vi "WaitForPolytecTrigger.vi"() -> (1 "Result":string)   [LabVIEW 2020]
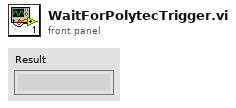
[diagram p1: front panel]
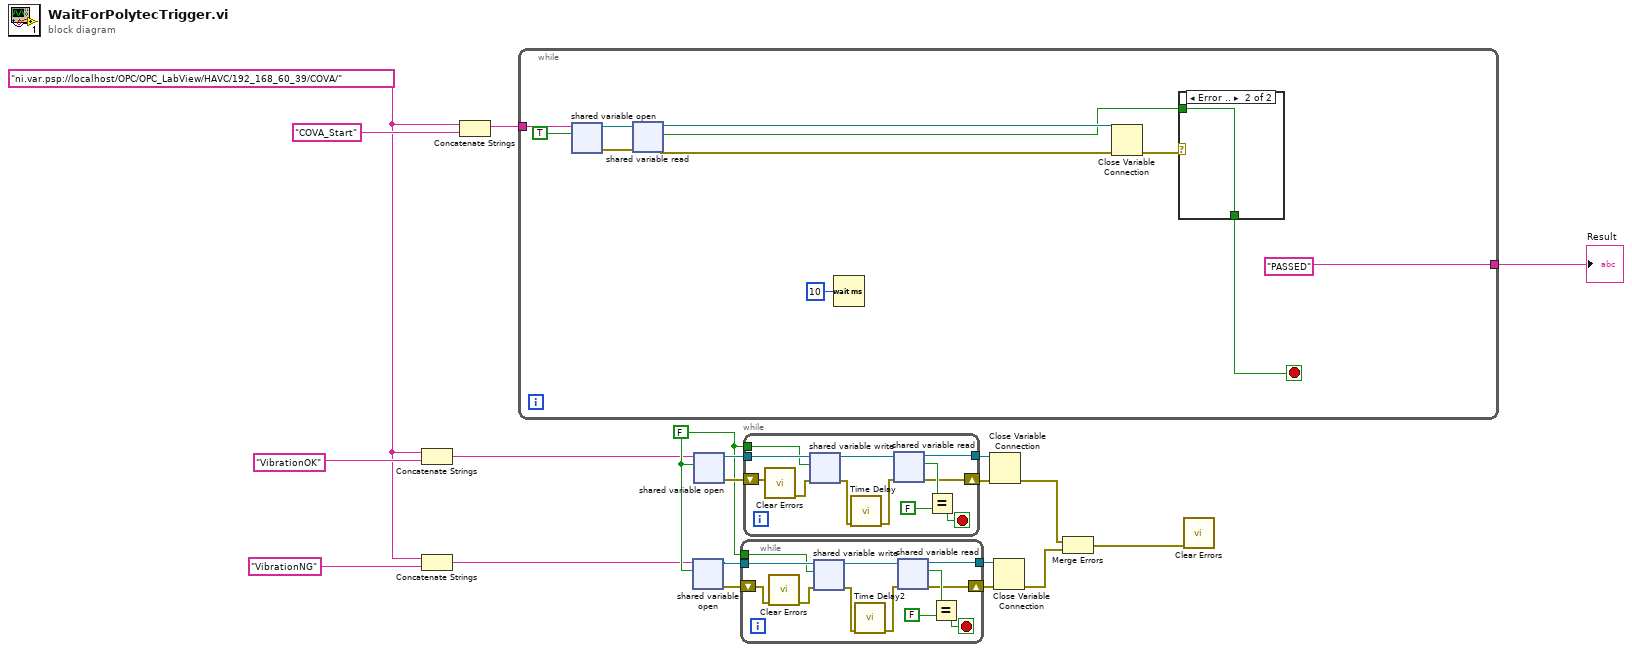
[diagram p0: block diagram]
diagram:
  w4 = FALSE
  w18 = "ni.var.psp://localhost/OPC/OPC_LabView/HAVC/192_168_60_39/COVA/" ("string")
  n1 = Concatenate Strings(w18, "VibrationOK") -> (w2:string)
  n2 = Concatenate Strings(w18, "VibrationNG" ("string")) -> (w3:string)
  n3 = Concatenate Strings(w18, "COVA_Start") -> (w16:string)
  n4 = while {
    tunnel: w16 -> [w31]
    tunnel: ["PASSED"] -> w15
    stop <- w24 stop-if-true
    n5 = shared-variable-open(w31, TRUE) -> (w28:refnum<k21>, w29:errorcluster)  [unwired: 2 in]
    n6 = shared-variable-read(w28, w29) -> (w26:refnum<k21>, w27:errorcluster, w23:bool)  [unwired: 1 out]
    n7 = Wait (ms)(milliseconds to wait=u32 10) -> ()  [unwired: 1 out]
    n8 = Close Variable Connection(8:w27, 11:w26) -> (0:w25:errorcluster)
    n9 = case shown="Error .." w25 {
      tunnel: [w32 w33] -> w24
      tunnel: w23 -> [w32 w33]
      frame No Error {
      }
      frame Error {
      }
    }
  }
  "Result" <- w15
  n10 = shared-variable-open(w3, w4) -> (w11:refnum<k21>, w12:errorcluster)  [unwired: 2 in]
  n11 = shared-variable-open(w2, w4) -> (w7:refnum<k21>, w14:errorcluster)  [unwired: 2 in]
  n12 = while {
    tunnel: [w40] -> w10
    tunnel: w11 -> [w39]
    tunnel: w4 -> [w35]
    shift-right: [w34] -> w13
    shift-left: w12 -> [w36]
    stop <- w38 stop-if-true
    n13 = call <vilib>:"Clear Errors.vi"("error in (no error)"=w36) -> ("error out"=w41:errorcluster)  [unwired: 5 in, 1 out]
    n14 = shared-variable-write(w39, w41, w35) -> (w43:refnum<k21>, w44:errorcluster)
    n15 = call "Time Delay2"("error in (no error)"=w44) -> ("error out"=w45:errorcluster)  [unwired: 10 in]
    n16 = shared-variable-read(w43, w45) -> (w40:refnum<k21>, w34:errorcluster, w37:bool)  [unwired: 1 out]
    n17 = Equal?(x=w37, y=FALSE) -> (x = y?=w38:bool)
  }
  n18 = while {
    tunnel: w7 -> [w54]
    tunnel: w4 -> [w53]
    tunnel: [w48] -> w9
    shift-right: [w49] -> w8
    shift-left: w14 -> [w46]
    stop <- w52 stop-if-true
    n19 = call <vilib>:"Clear Errors.vi"("error in (no error)"=w46) -> ("error out"=w47:errorcluster)  [unwired: 5 in, 1 out]
    n20 = shared-variable-write(w54, w47, w53) -> (w55:refnum<k21>, w56:errorcluster)
    n21 = call "Time Delay"("error in (no error)"=w56) -> ("error out"=w57:errorcluster)  [unwired: 10 in]
    n22 = shared-variable-read(w55, w57) -> (w48:refnum<k21>, w49:errorcluster, w51:bool)  [unwired: 1 out]
    n23 = Equal?(x=w51, y=FALSE) -> (x = y?=w52:bool)
  }
  n24 = Close Variable Connection(8:w8, 11:w9) -> (0:w6:errorcluster)
  n25 = Close Variable Connection(8:w13, 11:w10) -> (0:w5:errorcluster)
  n26 = Merge Errors(w6, w5) -> (w1:errorcluster)
  n27 = call <vilib>:"Clear Errors.vi"("error in (no error)"=w1) -> ()  [unwired: 5 in, 2 out]
